vi "Robot Main.vi"() -> ()   [LabVIEW 2018]
doc: "This VI implements the framework and scheduler for your robotics program. It should not be necessary to modify the framework. You are expected to add your code to the VIs called from Robot Main - the ones located in the Team Code folder within the project."
uses:
  <vilib>/Rock Robotics/WPI/Camera/WPI_CameraImageSize.ctl
  Robot Global Data.vi
panel:
  in  "Image Size":T1=enum."320x240"
  in  "Enable Vision":bool
  in  "Finish":bool
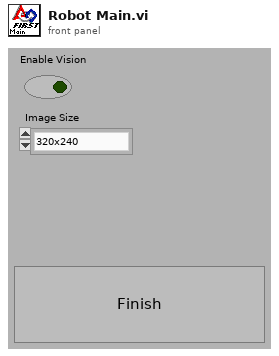
[diagram p1: front panel]
types:
  T1 = typedef "WPI_CameraImageSize.ctl" = enum16{"640x480", "320x240", "160x120", "Custom"}
  T2 = typedef "WPI_DriverStationMatch Info.ctl" = cluster{"Autonomous Elapsed Seconds":dbl, "TeleOp Elapsed Seconds":dbl, "Disabled Elapsed Seconds":dbl, "Visited Autonomous":bool, "Visited TeleOp":bool, "Visited Disabled":bool, "Autonomous Settings":cluster{"Autonomous Style":enum16{"Iterative", "Independent"}, "VI Refnum":refnum<vi>}}
  T3 = typedef "WPI_DriverStationDerivedRobotMode.ctl" = enum16{"Init", "Execute", "Stop"}
  T4 = typedef "WPI_DriverStationRobotMode2.ctl" = enum16{"Autonomous Disabled", "Autonomous Enabled", "Teleop Disabled", "Teleop Enabled", "Disconnected", "Finish", "Test Disabled", "Test Enabled", "Emergency Stopped"}
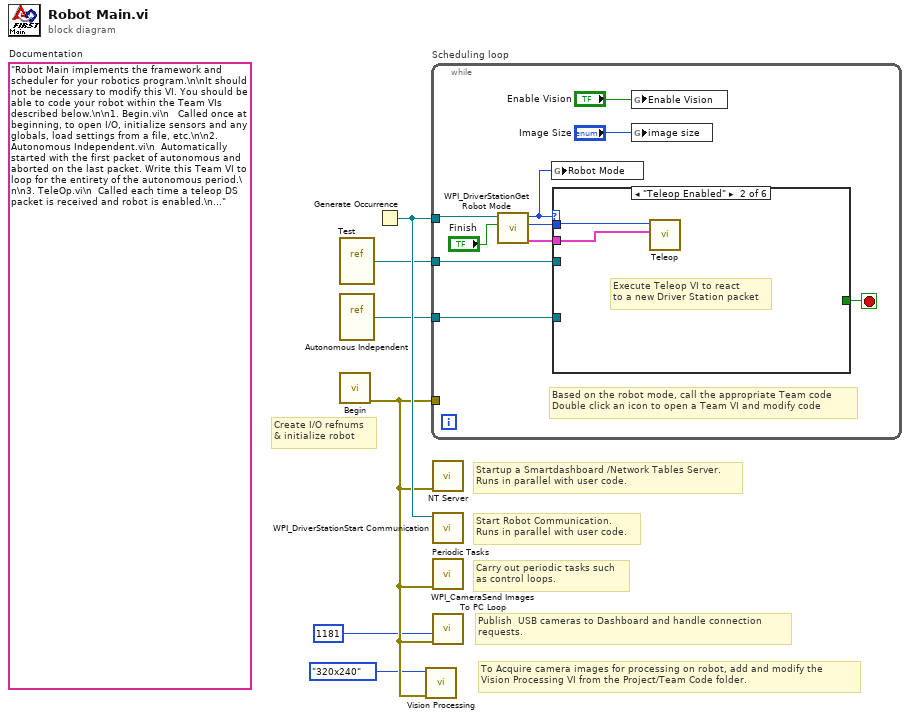
[diagram p0: block diagram]
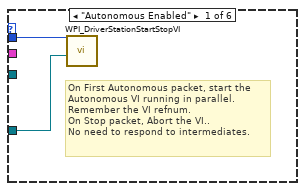
[diagram p2: hidden frame]
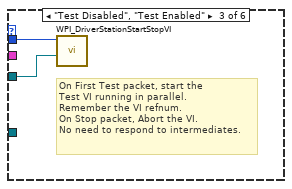
[diagram p3: hidden frame]
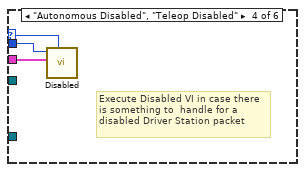
[diagram p4: hidden frame]
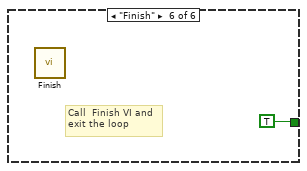
[diagram p6: hidden frame]
diagram:
  (unwired) "Robot Main implements the framework and scheduler for your robotics program.\n\nIt should not be necessary to modify this VI. You should be able to code your robot within the Team VIs described below.\n\n1. Begin.vi\n   Called once at beginning, to open I/O, initialize sensors and any globals, load settings from a file, etc.\n\n2. Autonomous Independent.vi\n  Automatically started with the first packet of autonomous and aborted on the last packet. Write this Team VI to loop for the entirety of the autonomous period.\n\n3. TeleOp.vi\n  Called each time a teleop DS packet is received and robot is enabled.\n\n4. Disabled.vi\n  Called each time a packet is received and the robot is disabled.\n\n5. Test.vi\n  Called Automatically started with the first test packet and aborted on the last. Modify this VI to carry out robot and sensor validation tests.\n\n6. Vision Processing.vi\n  A parallel loop that acquires and processes camera images. Drag from the project/Team Code if you wish to use this.\n\n7. PeriodicTasks.vi\n  Parallel loops running at user-defined rates.\n\n8. Finish.vi\n  Called before exiting, so you can save data, clean up I/O, etc.\n"  # Documentation
  # "Publish  USB cameras to Dashboard and handle connection\nrequests."
  # "Startup a Smartdashboard /Network Tables Server.\nRuns in parallel with user code."
  # "Carry out periodic tasks such\nas control loops."
  # "To Acquire camera images for processing on robot, add and modify the\nVision Processing VI from the Project/Team Code folder."
  # "Create I/O refnums\n& initialize robot"
  # "Start Robot Communication.\nRuns in parallel with user code."
  n1 = vi-ref "Test.vi"() -> (w4:refnum<vi>)
  n2 = vi-ref "Autonomous Independent.vi"() -> (w5:refnum<vi>)
  n3 = call "Begin.vi"() -> ("error out"=w3:errorcluster)  [unwired: 2 in, 9 out]
  n4 = Generate Occurrence() -> (w6:refnum<k4>)
  n5 = call "Vision Processing.vi"("error in (no error)"=w3, "Image Size"=WPI_CameraImageSize."320x240") -> ()  [unwired: 6 in]
  n6 = while "Scheduling loop" {
    tunnel: w6 -> [w15]
    tunnel: w3 -> [_]
    tunnel: w5 -> [w10]
    tunnel: w4 -> [w8]
    stop <- w12 stop-if-true
    # "Based on the robot mode, call the appropriate Team code\nDouble click an icon to open a Team VI and modify code"
    n7 = call <vilib>:"WPI_DriverStationGet Robot Mode.vi"("Finish"="Finish", "DS Occurrence"=w15) -> ("Match Info out"=w13:T2, "Call Context"=w16:T3, "Robot Mode"=w7:T4)  [unwired: 7 out]
    n8 = global write "Robot Global Data.vi" "Robot Mode"(w7) -> ()
    n9 = case shown="\"Teleop Enabled\"" w7 {
      selector: w7 -> [_ _ _ w23 _ _]
      tunnel: w16 -> [w18 w19 w22 w25 _ _]
      tunnel: w13 -> [_ w20 _ w24 _ _]
      tunnel: [_ _ _ _ _ TRUE] -> w12
      tunnel: w10 -> [w17 _ _ _ _ _]
      tunnel: w8 -> [_ _ w21 _ _ _]
      frame "Autonomous Enabled" {
        # "On First Autonomous packet, start the\nAutonomous VI running in parallel.\nRemember the VI refnum.\nOn Stop packet, Abort the VI..\nNo need to respond to intermediates."
        n10 = call <vilib>:"WPI_DriverStationStartStopVI.vi"("VI in"=w17, "Call Context"=w18) -> ()  [unwired: 10 in]
      }
      frame "Teleop Enabled" {
        # "Execute Teleop VI to react\nto a new Driver Station packet"
        n11 = call "Teleop.vi"("Match Info"=w20, "Call Context"=w19) -> ()  [unwired: 10 in]
      }
      frame "Test Disabled", "Test Enabled" {
        # "On First Test packet, start the\nTest VI running in parallel.\nRemember the VI refnum.\nOn Stop packet, Abort the VI.\nNo need to respond to intermediates."
        n12 = call <vilib>:"WPI_DriverStationStartStopVI.vi"("VI in"=w21, "Call Context"=w22) -> ()  [unwired: 10 in]
      }
      frame "Autonomous Disabled", "Teleop Disabled" {
        # "Execute Disabled VI in case there\nis something to  handle for a\ndisabled Driver Station packet"
        n13 = call "Disabled.vi"("Robot Mode"=w23, "Match Info"=w24, "Call Context"=w25) -> ()  [unwired: 1 in, 8 out]
      }
      frame "Disconnected", Default {
        # "Driver Station packet didn't arrive.\nPossibly useful for diagnostics"
      }
      frame "Finish" {
        # "Call  Finish VI and\nexit the loop"
        n14 = call "Finish.vi"() -> ()  [unwired: 1 in, 7 out]
      }
    }
    n15 = global write "Robot Global Data.vi" "Enable Vision"("Enable Vision") -> ()
    n16 = global write "Robot Global Data.vi" "image size"("Image Size") -> ()
  }
  n17 = call <vilib>:"NT Server.vi"("error in (no error)"=w3) -> ()  [unwired: 11 in]
  n18 = call <vilib>:"WPI_DriverStationStart Communication.vi"("occurrence"=w6) -> ()  [unwired: 1 in, 10 out]
  n19 = call "Periodic Tasks.vi"("error in"=w3) -> ()  [unwired: 1 in, 10 out]
  n20 = call <vilib>:"WPI_CameraSend Images To PC Loop.vi"("error in (no error)"=w3, "port"=u16 1181) -> ()  [unwired: 10 in]
